vi "PAN_CheckSave.vi"(10 "cmd in":string) -> ()   [LabVIEW 2016]
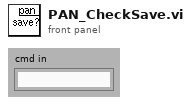
[diagram p1: front panel]
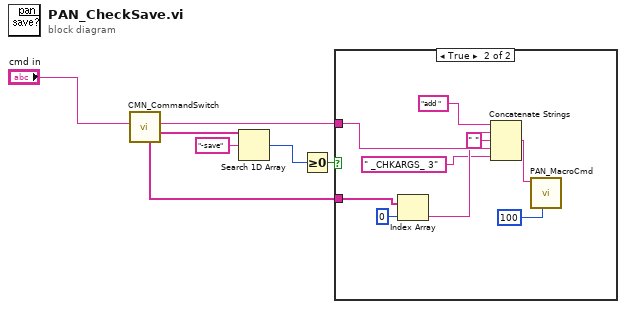
[diagram p0: block diagram]
diagram:
  n1 = call "CMN_CommandSwitch.vi"("command in"="cmd in") -> ("swhitches"=w6:string[], "command out"=w1:string, "arguments"=w2:string[])  [unwired: 1 in, 7 out]
  n2 = Search 1D Array(1D array=w6, element="-save") -> (index of element=w4:i32)  [unwired: 1 out]
  n3 = Greater Or Equal To 0?(x=w4) -> (x >= 0?=w3:bool)
  n4 = case shown="True" w3 {
    tunnel: w2 -> [_ w16]
    tunnel: w1 -> [_ w12]
    frame False {
    }
    frame True {
      n5 = Index Array(array=w16, index=0) -> (element=w11:string)
      n6 = Concatenate Strings("add " ("string"), w11, " " ("string"), w12, " _CHKARGS_ 3" ("string")) -> (w13:string)
      n7 = call "PAN_MacroCmd.vi"("timeout in ms (-1)"=100, "Command"=w13) -> ()  [unwired: 1 in, 9 out]
    }
  }
